vi "UMLEditor_GraphMemory.vi"(0 "GraphIn":refnum<class "Graph.lvclass">, 2 "error in (no error)":errorcluster) -> (14 "GraphOut":refnum<class "Graph.lvclass">, 16 "error out":errorcluster)   [LabVIEW 2012]
doc: "This VI is used to manage system paths.\n\nName: The name of the path to be set or retrieved. The default Name is Home.\n\nPath In: Used to specify the path for Set Path method.\n\nPath Out: Returns the path for Get Path method.\n\nerror out: Returns error info if appropriate.\n\nMethod: {Get Path, Set Path, Delete Path, Clear All Paths}\n\nAuthor: SPCase\nCopyright 2003 VI Engineering, Inc.\n\nCurrent Revision: 12\nVSS Version: 2"
uses:
  <resource>/Framework/Providers/Open_GDS/UML/Graph_class/Graph.lvclass
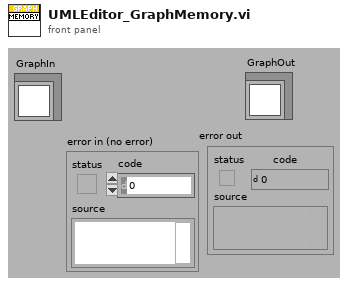
[diagram p1: front panel]
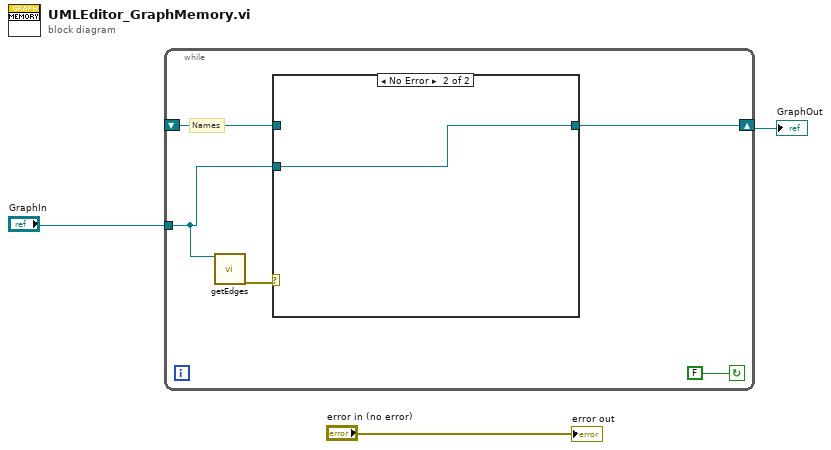
[diagram p0: block diagram]
diagram:
  n1 = while {
    shift-left: _ -> [w7]
    shift-right: [w6] -> w1
    tunnel: "GraphIn" -> [w5]
    stop <- FALSE continue-if-true
    # "Names"
    n2 = call-dynamic "getEdges.vi"("reference"=w5) -> ("error out"=w4:errorcluster)  [unwired: 16 in, 2 out]
    n3 = case shown="No Error" w4 {
      tunnel: w7 -> [w9 _]
      tunnel: [w9 w10] -> w6
      tunnel: w5 -> [_ w10]
      frame Error {
      }
      frame No Error {
      }
    }
  }
  "GraphOut" <- w1
  "error out" <- "error in (no error)"
